vi "test Disconnect All.vi"(8 "error in (no error)":errorcluster, 11 "TestCase in":refnum<class "SLSC Switch Messaging Tests.lvclass">) -> (0 "error out":errorcluster, 3 "TestCase out":refnum<class "SLSC Switch Messaging Tests.lvclass">)   [LabVIEW 2020, in "SLSC Switch Messaging Tests.lvclass"]
uses:
  SLSC Switch Messaging Tests.lvclass
  Includes/CDMessaging.lvlibp/Switch/Switch Disconnect All Message/Switch Disconnect All Message.lvclass
  C:/Users/nitest/Desktop/Git 2020/niveristand-routing-and-faulting-message-library/Includes/CDMessaging.lvlibp/Message/Abstract Message/Abstract Message.lvclass
  Support/Mock SLSC Switch Consumer.lvclass
  SLSC Switch Messaging Tests.lvclass/SLSC Switch Messaging Tests.ctl
  Support/Mock SLSC Switch Consumer.lvclass/Mock SLSC Switch Consumer.ctl
  Support/Read Connections.vi
  Includes/CDMessaging.lvlibp/Switch/Abstract Switch Consumer/Abstract Switch Consumer.lvclass
  C:/Users/nitest/Desktop/Git 2020/niveristand-routing-and-faulting-message-library/Includes/CDMessaging.lvlibp/Consumer/Abstract Consumer/Abstract Consumer.lvclass
  Includes/CDMessaging.lvlibp/Producer/Abstract Producer/Abstract Producer.lvclass
  <vilib>/addons/_JKI Toolkits/VI Tester/TestCase.llb/TestCase.lvclass
  Includes/CDMessaging.lvlibp/Consumer/Abstract Consumer/Abstract Consumer.lvclass
  C:/Program Files (x86)/National Instruments/LabVIEW 2020/vi.lib/addons/_JKI Toolkits/VI Tester/TestCase.llb/TestCase.lvclass
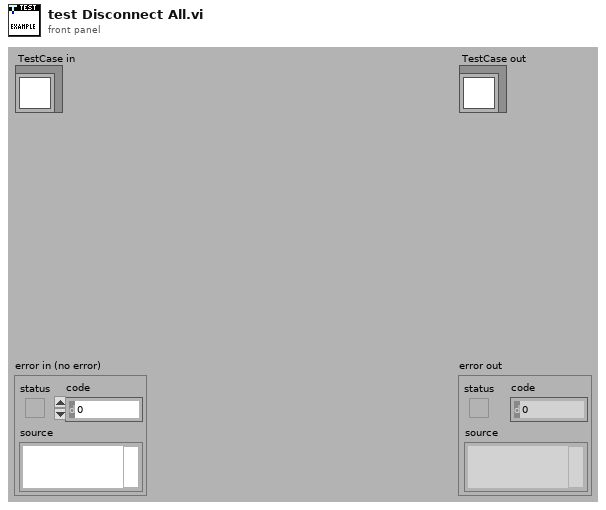
[diagram p1: front panel]
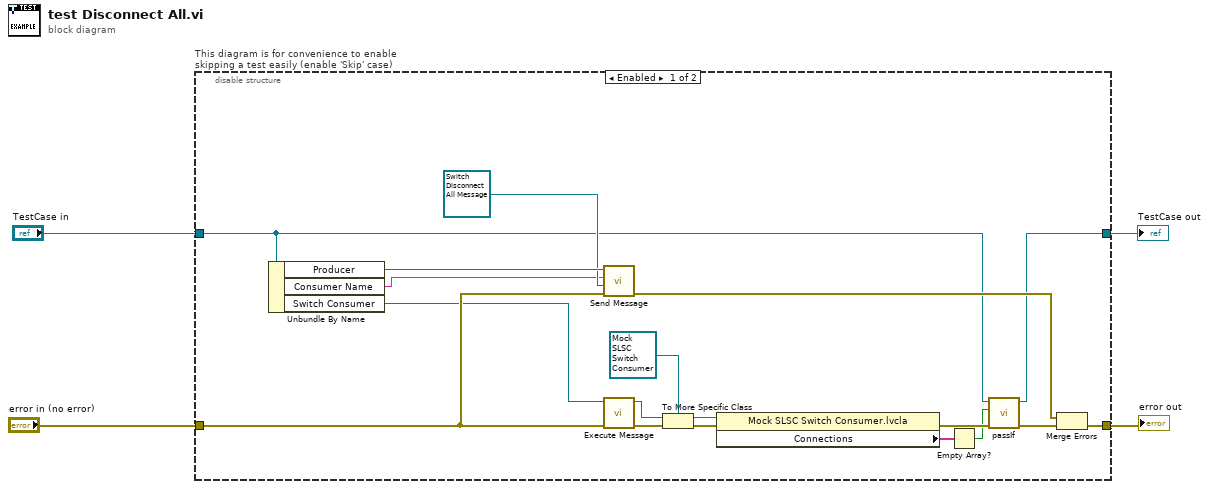
[diagram p0: block diagram]
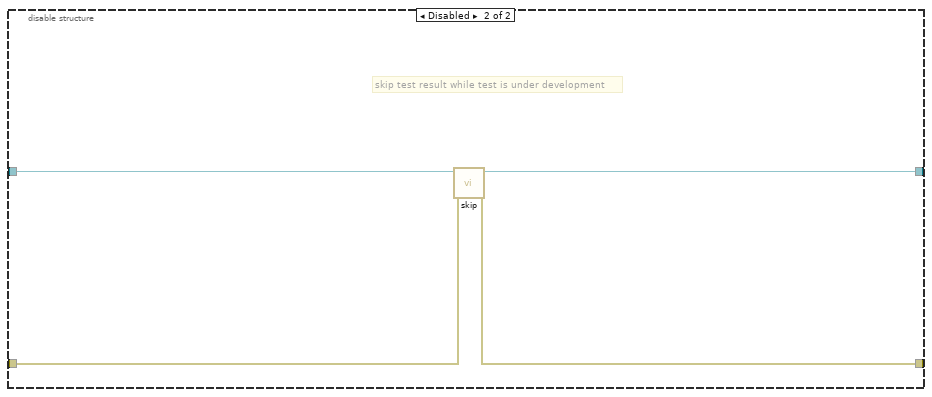
[diagram p2: hidden frame]
diagram:
  n1 = disable-structure "This diagram is for convenience to enable skipping a test easily (enable 'Skip' case)" shown="Enabled" {
    disable-tunnel: "TestCase in" -> [w9 w26]
    disable-tunnel: [w8 w24] -> w1
    disable-tunnel: [w16 w25] -> w3
    disable-tunnel: "error in (no error)" -> [w19 w23]
    frame Enabled {
      n2 = Unbundle By Name(w9) -> ("Producer"=w22:refnum<class "Abstract Producer.lvclass">, "Consumer Name"=w20:string, "Switch Consumer"=w18:refnum<class "Abstract Switch Consumer.lvclass">)
      n3 = call-dynamic "Send Message.vi"("error in (no error)"=w19, "Message in"=refnum<class "Switch Disconnect All Message.lvclass"> refnum ("CDMessaging.lvlibp:Switch Disconnect All Message.lvclass"), "Consumer in"=w20, "Abstract Producer in"=w22) -> ("error out"=w17:errorcluster)  [unwired: 4 in, 3 out]
      n4 = call "Execute Message.vi"("error in (no error)"=w19, "Abstract Consumer in"=w18) -> ("error out"=w15:errorcluster, "Abstract Consumer out"=w14:refnum<class "Abstract Consumer.lvclass">)  [unwired: 6 in, 2 out]
      n5 = To More Specific Class(target class=refnum<class "Mock SLSC Switch Consumer.lvclass"> refnum ("Mock SLSC Switch Consumer.lvclass"), reference=w14, error in=w15) -> (specific class reference=w12:refnum<class "Mock SLSC Switch Consumer.lvclass">, error out=w11:errorcluster)
      n6 = property class="Mock SLSC Switch Consumer.lvcla"(reference=w12, error in=w11) -> (error out=w10:errorcluster, "Connections"=w6:string[])  [unwired: 1 out]
      n7 = Empty Array?(array=w6) -> (empty?=w5:bool)
      n8 = call-dynamic "passIf.vi"("error in (no error)"=w10, "pass"=w5, "TestCase in"=w9) -> ("error out"=w7:errorcluster, "TestCase out"=w8:refnum<class "SLSC Switch Messaging Tests.lvclass">)  [unwired: 7 in]
      n9 = Merge Errors(w17, w7) -> (w16:errorcluster)
    }
    frame Disabled {
      # "skip test result while test is under development"
      n10 = call <vilib>:"skip.vi"("error in (no error)"=w23, "TestCase in"=w26) -> ("error out"=w25:errorcluster, "TestCase out"=w24:refnum<class "SLSC Switch Messaging Tests.lvclass">)  [unwired: 8 in]
    }
  }
  "error out" <- w3
  "TestCase out" <- w1
